vi "Update Status Channels.vi"(4 "Finished Late? [i-1]":bool, 6 "Iteration Duration":i64, 8 "error in (no error)":errorcluster, 11 "Engine Run Time Data in":T1) -> (0 "error out":errorcluster, 3 "Engine Run Time Data out":T1)   [LabVIEW 2023, in "NI 272x Resistive Simulation Custom Device Engine.lvlib"]
uses:
  NI 272x Resistive Simulation Custom Device Engine.lvlib
  Controls/Engine Run Time Data.ctl
  Controls/Compiled Engine Data.ctl
  Controls/Compiled HW Channel.ctl
  Controls/Channel Mode.ctl
  <instrlib>/ni272xReferenceVIs/ni272xReferenceVIs.llb/ni272x Callendar-Van Dusen RTD Parameters.ctl
  Controls/Compiled Connect Channel.ctl
  <instrlib>/ni272xReferenceVIs/ni272xReferenceVIs.llb/ni272x Reference.ctl
  NI 272x Resistive Simulation Custom Device Shared.lvlib
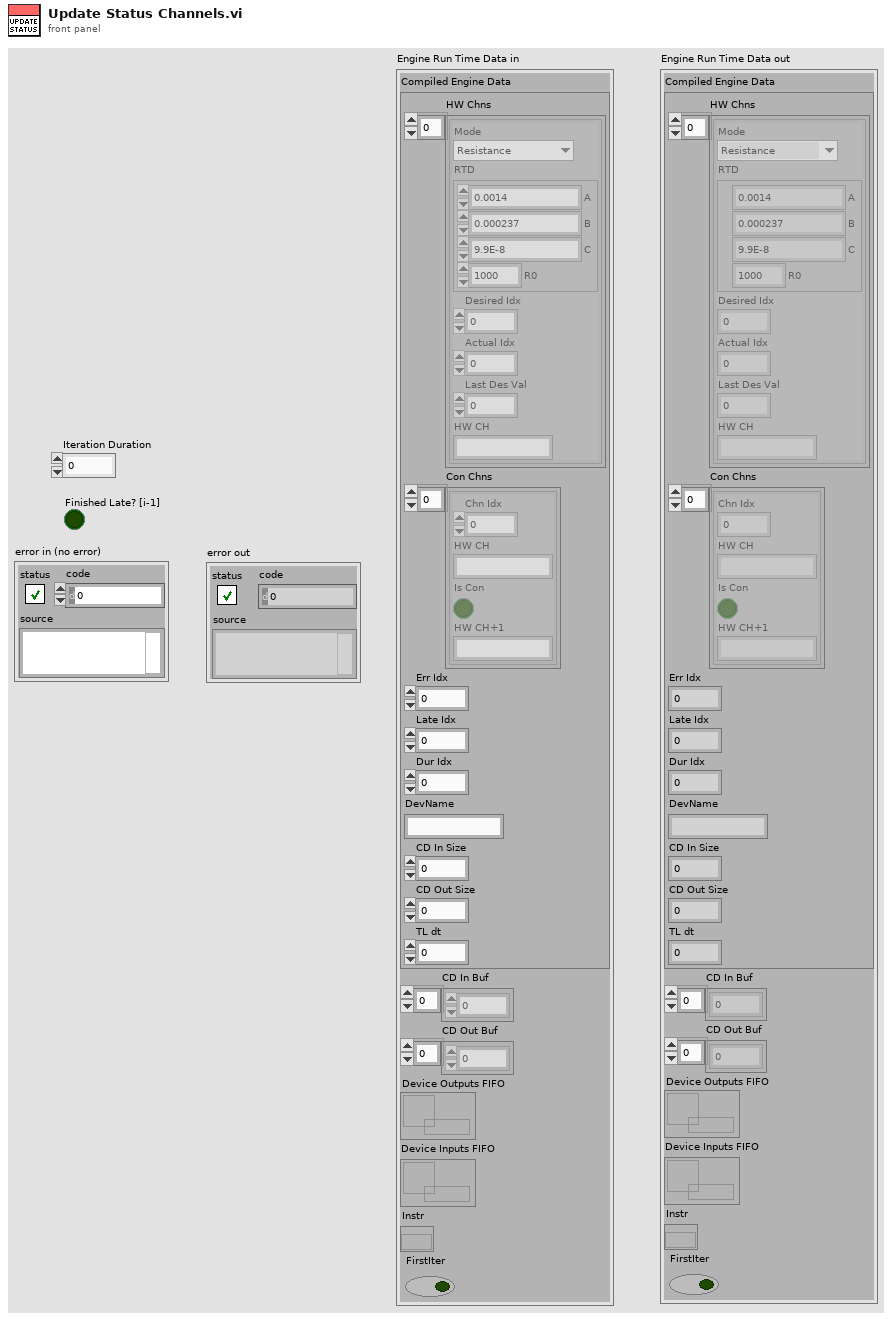
[diagram p1: front panel]
types:
  T1 = typedef "NI 272x Resistive Simulation Custom Device Engine.lvlib/Engine Run Time Data.ctl" = cluster{"Compiled Engine Data":T2, "CD In Buf":dbl[], "CD Out Buf":dbl[], "Device Outputs FIFO":refnum<k33>, "Device Inputs FIFO":refnum<k33>, "Instr":T7, "FirstIter":bool}
  T2 = typedef "NI 272x Resistive Simulation Custom Device Shared.lvlib/Compiled Engine Data.ctl" = cluster{"HW Chns":T3[], "Con Chns":T6[], "Err Idx":i32, "Late Idx":i32, "Dur Idx":i32, "DevName":string, "CD In Size":i32, "CD Out Size":i32, "TL dt":i64}
  T3 = typedef "NI 272x Resistive Simulation Custom Device Shared.lvlib/Compiled HW Channel.ctl" = cluster{"Mode":T4, "RTD":T5, "Desired Idx":i32, "Actual Idx":i32, "Last Des Val":dbl, "HW CH":string}
  T4 = typedef "NI 272x Resistive Simulation Custom Device Shared.lvlib/Channel Mode.ctl" = enum16{"Resistance", "RTD Temperature"}
  T5 = typedef "ni272x Callendar-Van Dusen RTD Parameters.ctl" = cluster{"A":dbl, "B":dbl, "C":dbl, "R0":dbl}
  T6 = typedef "NI 272x Resistive Simulation Custom Device Shared.lvlib/Compiled Connect Channel.ctl" = cluster{"Chn Idx":i32, "HW CH":string, "Is Con":bool, "HW CH+1":string}
  T7 = typedef "ni272x Reference.ctl" = refnum<k20>
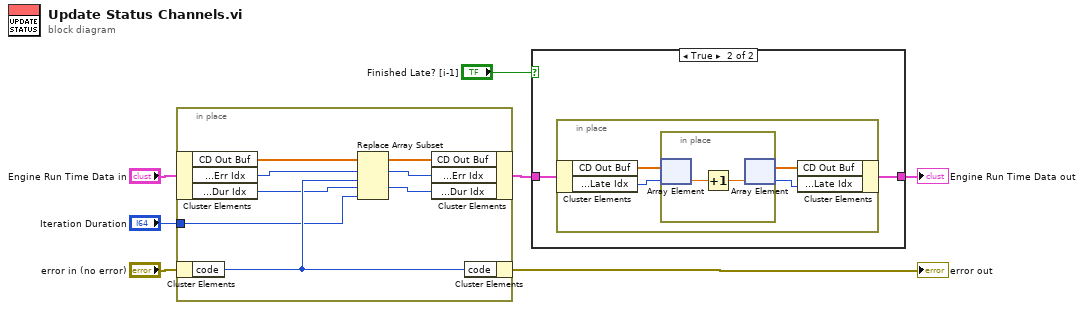
[diagram p0: block diagram]
diagram:
  n1 = in-place {
    in-place-border: "Iteration Duration" -> [w9]
    n2 = in-place-cluster #1("Engine Run Time Data in") -> ("CD Out Buf"=w13:dbl[], "Compiled Engine Data.Err Idx"=w11:i32, "Compiled Engine Data.Dur Idx"=w8:i32)
    n3 = in-place-cluster #2("error in (no error)") -> ("code"=w10:i32)
    n4 = Replace Array Subset(array=w13, new element #1=w10, index #1=w11, new element #2=w9, index #2=w8) -> (w12:dbl[])
    n5 = in-place-cluster #1("CD Out Buf"=w12, "Compiled Engine Data.Err Idx"=w11, "Compiled Engine Data.Dur Idx"=w8) -> (w3:T1)
    n6 = in-place-cluster #2("code"=w10) -> (→"error out":errorcluster)
  }
  n7 = case shown="True" "Finished Late? [i-1]" {
    tunnel: w3 -> [w14 w16]
    tunnel: [w14 w15] -> w1
    frame False {
    }
    frame True {
      n8 = in-place {
        n9 = in-place-cluster #3(w16) -> ("CD Out Buf"=w20:dbl[], "Compiled Engine Data.Late Idx"=w19:i32)
        n10 = in-place {
          n11 = in-place-array #4(w20, w19) -> (w22:dbl)
          n12 = Increment(x=w22) -> (x+1=w21:dbl)
          n13 = in-place-array #4(w21) -> (w18:dbl[], w17:i32)
        }
        n14 = in-place-cluster #3("CD Out Buf"=w18, "Compiled Engine Data.Late Idx"=w17) -> (w15:T1)
      }
    }
  }
  "Engine Run Time Data out" <- w1
